vi "Read Display Format.vi"(9 "NumericText in":refnum<class "Digital.lvclass">) -> (3 "NumericText out":refnum<class "Digital.lvclass">, 4 "Display Format":T1)   [LabVIEW 2014, in "Digital.lvclass"]
uses:
  Digital.lvclass
  <vilib>/Utility/miscctls.llb/LVFormatAndPrecisionTypeDef.ctl
  Digital.lvclass/Digital.ctl
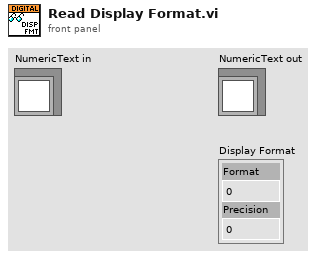
[diagram p1: front panel]
types:
  T1 = typedef "LVFormatAndPrecisionTypeDef.ctl" = cluster{"Format":u8, "Precision":u8}
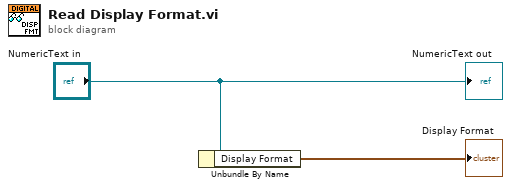
[diagram p0: block diagram]
diagram:
  n1 = Unbundle By Name("NumericText in") -> ("Display Format"=→"Display Format":T1)
  "NumericText out" <- "NumericText in"
